vi "Deliver Result.vi"(8 "error in (no error)":errorcluster, 10 "result":refnum<class "result.lvclass">, 11 "input_poller_queue in":refnum<class "input_poller_queue.lvclass">) -> (0 "error out":errorcluster, 3 "input_poller_queue out":refnum<class "input_poller_queue.lvclass">)   [LabVIEW 2015, in "input_poller_queue.lvclass"]
uses:
  input_poller_queue.lvclass
  Result/result.lvclass
  input_poller_queue.lvclass/input_poller_queue.ctl
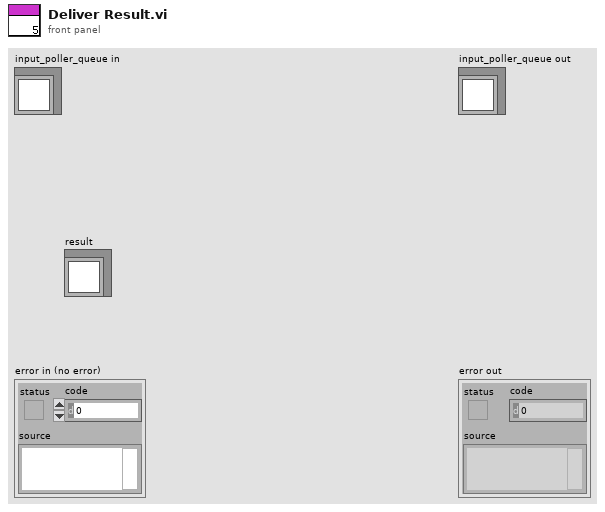
[diagram p1: front panel]
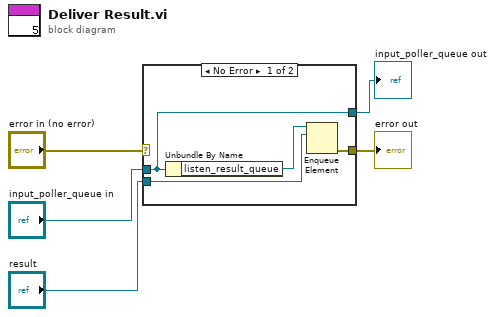
[diagram p0: block diagram]
diagram:
  n1 = case shown="No Error" "error in (no error)" {
    selector: "error in (no error)" -> [_ w11]
    tunnel: [w7 w11] -> w4
    tunnel: [w6 w10] -> w3
    tunnel: "input_poller_queue in" -> [w6 w10]
    tunnel: "result" -> [w8 _]
    frame No Error {
      n2 = Unbundle By Name(w6) -> ("listen_result_queue"=w9:refnum<queue>)
      n3 = Enqueue Element(queue=w9, element=w8) -> (error out=w7:errorcluster)  [unwired: 2 in, 2 out]
    }
    frame Error {
    }
  }
  "error out" <- w4
  "input_poller_queue out" <- w3
